vi "TCP Command Parse.vi"(1 "Command Msg":string) -> (6 "PXI6123_CH_ON":i32[](array[ring]) items=["OFF", "ON"], 7 "PXI6254_CH_ON":i32[](array[ring]) items=["OFF", "ON"], 9 "TestTime":dbl, 10 "PXI6122_CH_ON":i32[](array[ring]) items=["OFF", "ON"], 11 "PXI6733_CH_OFFSET":dbl[](array[numeric]) min=0.0 max=1000000.0 step=0.001, 13 "PXI6733_CH_FREQ":dbl[](array[numeric]) min=1e-06 max=1000000.0 step=0.1, 15 "PXI6733_CH_ON":i32[](array[ring]) items=["OFF", "ON"], 17 "PXI6733_CH_WAVE":i32[](array[ring])=[1, 1, 1, 1, 1, 1, 1, 1] items=["SIN_WAVW"=1, "SQUARE_WAVE"=2, "TRI_WAVE"=3, "CONST_WAVE"=4, "PROP_WAVE"=5, "WRITE_NOISE"=6], 18 "PXI6733_CH_AMP":dbl[](array[numeric]) min=0.0 max=1000000.0 step=0.001)   [LabVIEW 2011]
doc: "Reads an incoming package of data from a remote host via TCP/IP. This VI parses the package and extracts the data name and type as described in the meta data.\n\nFor the package to be parsed correctly, the meta data must be consistent in both the sender and the receiver. The data is packaged based on the existing meta data on the sender. Inconsistent meta data will result in inconsistent data parsing.\nUse the \"Read Meta\" and \"Write Meta\" VIs to ensure that both client and server have the same meta data.\n\nThe data is returned as a string. It is the responsibility of the user to cast it to the appropriate type before usage."
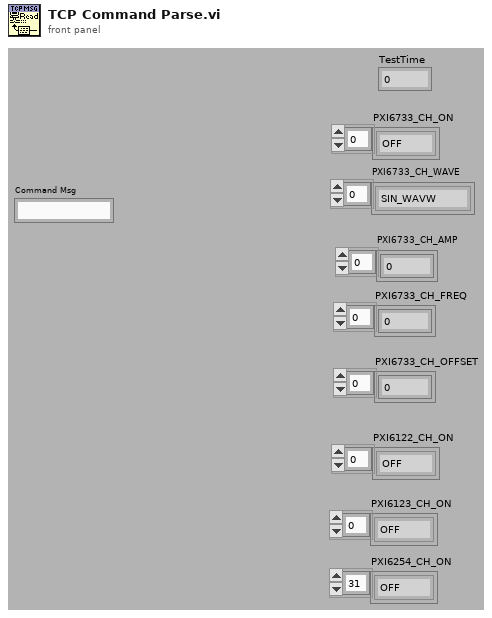
[diagram p1: front panel]
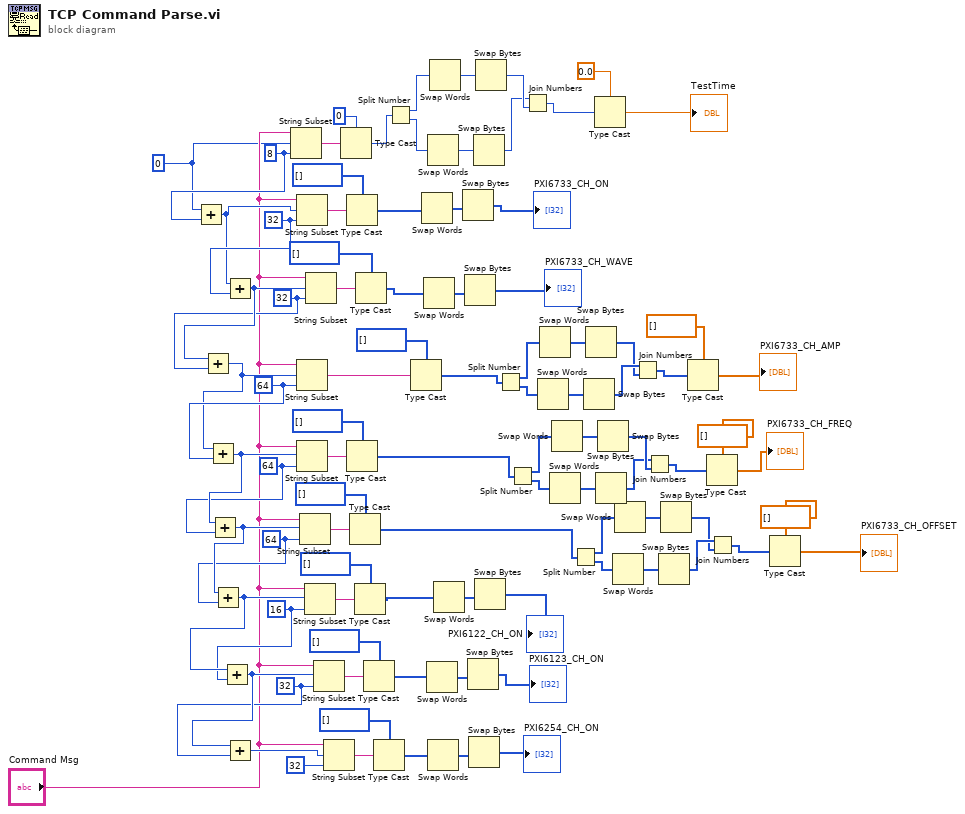
[diagram p0: block diagram]
diagram:
  w1 = 0 ("x")
  w59 = 32 ("length (rest)")
  w70 = 32 ("length (rest)")
  w64 = 16 ("length (rest)")
  w76 = 64 ("length (rest)")
  w80 = 64 ("length (rest)")
  w84 = 64 ("length (rest)")
  w73 = 32 ("length (rest)")
  w68 = 8 ("length (rest)")
  n1 = Add(x=w1, y=w68) -> (x+y=w69:i32)
  n2 = Add(x=w69, y=w73) -> (x+y=w71:i32)
  n3 = Add(x=w71, y=w70) -> (x+y=w72:i32)
  n4 = Add(x=w72, y=w84) -> (x+y=w81:i32)
  n5 = Add(x=w81, y=w80) -> (x+y=w77:i32)
  n6 = Add(x=w77, y=w76) -> (x+y=w65:i32)
  n7 = Add(x=w65, y=w64) -> (x+y=w60:i32)
  n8 = Add(x=w60, y=w59) -> (x+y=w58:i32)
  n9 = String Subset(string="Command Msg", offset (0)=w1, length (rest)=w68) -> (substring=w92:string)
  n10 = String Subset(string="Command Msg", offset (0)=w69, length (rest)=w73) -> (substring=w90:string)
  n11 = String Subset(string="Command Msg", offset (0)=w72, length (rest)=w84) -> (substring=w87:string)
  n12 = String Subset(string="Command Msg", offset (0)=w81, length (rest)=w80) -> (substring=w86:string)
  n13 = String Subset(string="Command Msg", offset (0)=w77, length (rest)=w76) -> (substring=w82:string)
  n14 = String Subset(string="Command Msg", offset (0)=w65, length (rest)=w64) -> (substring=w79:string)
  n15 = String Subset(string="Command Msg", offset (0)=w71, length (rest)=w70) -> (substring=w75:string)
  n16 = String Subset(string="Command Msg", offset (0)=w60, length (rest)=w59) -> (substring=w66:string)
  n17 = String Subset(string="Command Msg", offset (0)=w58, length (rest)=32 ("length (rest)")) -> (substring=w63:string)
  n18 = Type Cast(type=i64 0 ("bytes to read"), x=w92) -> (*(type *) &x=w36:i64)
  n19 = Type Cast(type=i32[] [], x=w90) -> (*(type *) &x=w57:i32[])
  n20 = Type Cast(type=i64[] [], x=w86) -> (*(type *) &x=w16:i64[])
  n21 = Type Cast(type=i64[] [], x=w82) -> (*(type *) &x=w5:i64[])
  n22 = Type Cast(type=i32[] [], x=w79) -> (*(type *) &x=w50:i32[])
  n23 = Type Cast(type=i32[] [], x=w75) -> (*(type *) &x=w54:i32[])
  n24 = Type Cast(type=i32[] [], x=w66) -> (*(type *) &x=w47:i32[])
  n25 = Type Cast(type=i32[] [], x=w63) -> (*(type *) &x=w44:i32[])
  n26 = Split Number(x=w36) -> (hi(x)=w41:u32, lo(x)=w39:u32)
  n27 = Type Cast(type=i64[] [], x=w87) -> (*(type *) &x=w26:i64[])
  n28 = Swap Words(1:w57) -> (0:w56:i32[])
  n29 = Swap Words(1:w54) -> (0:w53:i32[])
  n30 = Swap Words(1:w47) -> (0:w48:i32[])
  n31 = Swap Words(1:w39) -> (0:w40:u32)
  n32 = Swap Words(1:w44) -> (0:w45:i32[])
  n33 = Swap Words(1:w41) -> (0:w42:u32)
  n34 = Swap Words(1:w50) -> (0:w51:i32[])
  n35 = Swap Bytes(anything=w56) -> (byte swapped=→"PXI6733_CH_ON":i32[])
  n36 = Swap Bytes(anything=w53) -> (byte swapped=→"PXI6733_CH_WAVE":i32[])
  n37 = Swap Bytes(anything=w48) -> (byte swapped=→"PXI6123_CH_ON":i32[])
  n38 = Swap Bytes(anything=w45) -> (byte swapped=→"PXI6254_CH_ON":i32[])
  n39 = Swap Bytes(anything=w40) -> (byte swapped=w37:u32)
  n40 = Swap Bytes(anything=w51) -> (byte swapped=→"PXI6122_CH_ON":i32[])
  n41 = Swap Bytes(anything=w42) -> (byte swapped=w38:u32)
  n42 = Split Number(x=w26) -> (hi(x)=w28:u32[], lo(x)=w30:u32[])
  n43 = Split Number(x=w16) -> (hi(x)=w21:u32[], lo(x)=w19:u32[])
  n44 = Join Numbers(hi=w37, lo=w38) -> ((hi.lo)=w35:u64)
  n45 = Swap Words(1:w30) -> (0:w29:u32[])
  n46 = Swap Words(1:w28) -> (0:w27:u32[])
  n47 = Swap Words(1:w19) -> (0:w20:u32[])
  n48 = Swap Words(1:w21) -> (0:w22:u32[])
  n49 = Split Number(x=w5) -> (hi(x)=w7:u32[], lo(x)=w9:u32[])
  n50 = Swap Bytes(anything=w29) -> (byte swapped=w32:u32[])
  n51 = Swap Bytes(anything=w27) -> (byte swapped=w31:u32[])
  n52 = Type Cast(type=0.0 ("bytes to read"), x=w35) -> (*(type *) &x=→"TestTime":dbl)
  n53 = Swap Bytes(anything=w20) -> (byte swapped=w17:u32[])
  n54 = Swap Bytes(anything=w22) -> (byte swapped=w18:u32[])
  n55 = Swap Words(1:w9) -> (0:w8:u32[])
  n56 = Swap Words(1:w7) -> (0:w6:u32[])
  n57 = Join Numbers(hi=w32, lo=w31) -> ((hi.lo)=w25:u64[])
  n58 = Join Numbers(hi=w17, lo=w18) -> ((hi.lo)=w15:u64[])
  n59 = Swap Bytes(anything=w8) -> (byte swapped=w11:u32[])
  n60 = Swap Bytes(anything=w6) -> (byte swapped=w10:u32[])
  n61 = Type Cast(type=dbl[] [], x=w25) -> (*(type *) &x=→"PXI6733_CH_AMP":dbl[])
  n62 = Type Cast(type=dbl[] [], x=w15) -> (*(type *) &x=→"PXI6733_CH_FREQ":dbl[])
  n63 = Join Numbers(hi=w11, lo=w10) -> ((hi.lo)=w12:u64[])
  n64 = Type Cast(type=dbl[] [], x=w12) -> (*(type *) &x=→"PXI6733_CH_OFFSET":dbl[])
